vi "Rodrigues.vi"   [LabVIEW 2020, in "g_ar_toolkit.ar.lvlib"]
uses:
  g_ar_toolkit.ar.lvlib
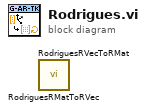
[diagram p0: block diagram]
diagram:
  n1 = call "RodriguesRMatToRVec.vi"() -> ()  [unwired: 10 in, 2 out]
  n2 = call "RodriguesRVecToRMat.vi"() -> ()  [unwired: 10 in, 2 out]
